vi "Test Process Error on Request Propagated to Caller.vi"(8 "error in (no error)":errorcluster, 11 "Process Test In":refnum<class "Process Dev Test.lvclass">) -> (0 "error out":errorcluster, 3 "Process Test Out":refnum<class "Process Dev Test.lvclass">)   [LabVIEW 2020, in "Process Dev Test.lvclass"]
uses:
  Process Dev Test.lvclass
  Process Dev Test.lvclass/Process Dev Test.ctl
  source/Framework Test Suite/Mock Process/Mock Process.lvclass
  source/Framework/Process/Process.lvclass
  <vilib>/ErrorRing/Error Ring.xnode
  <vilib>/Utility/error.llb/Error Cluster From Error Code.vi
  C:/Git/triarc-framework/source/Framework/Process/Process.lvclass
  C:/Git/triarc-framework/source/Framework/Base/Base.lvclass
  C:/Git/triarc-framework/source/Framework/Configuration File/Configuration File.lvclass
  C:/Git/triarc-framework/source/Framework/Configuration/Configuration.lvclass
  C:/Git/triarc-framework/source/Framework/Error Handler Interface/Error Handler Interface.lvclass
  C:/Git/triarc-framework/source/Framework/Logging/Logging.lvclass
  C:/Git/triarc-framework/source/Framework Test Suite/Mock Process/Mock Process.lvclass
  C:/Git/triarc-framework/source/Framework/Async Handler/Async Handler.lvclass
  C:/Git/triarc-framework/source/Framework/Helper Loop/Helper Loop.lvclass
  <vilib>/Astemes/LUnit/Test Case.lvclass
  C:/Git/triarc-framework/source/Framework Test Suite/Base Class Test/Base Test.lvclass
  C:/Program Files (x86)/National Instruments/LabVIEW 2020/vi.lib/Astemes/LUnit/Test Case.lvclass
  C:/Git/triarc-framework/tests/Process Development Test/Process Test/Process Dev Test.lvclass
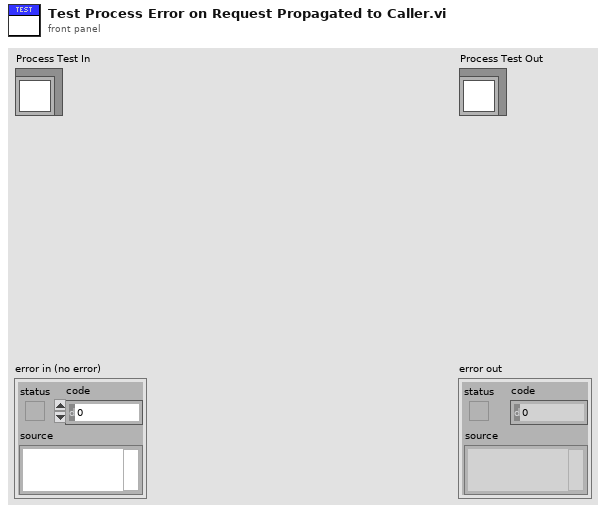
[diagram p1: front panel]
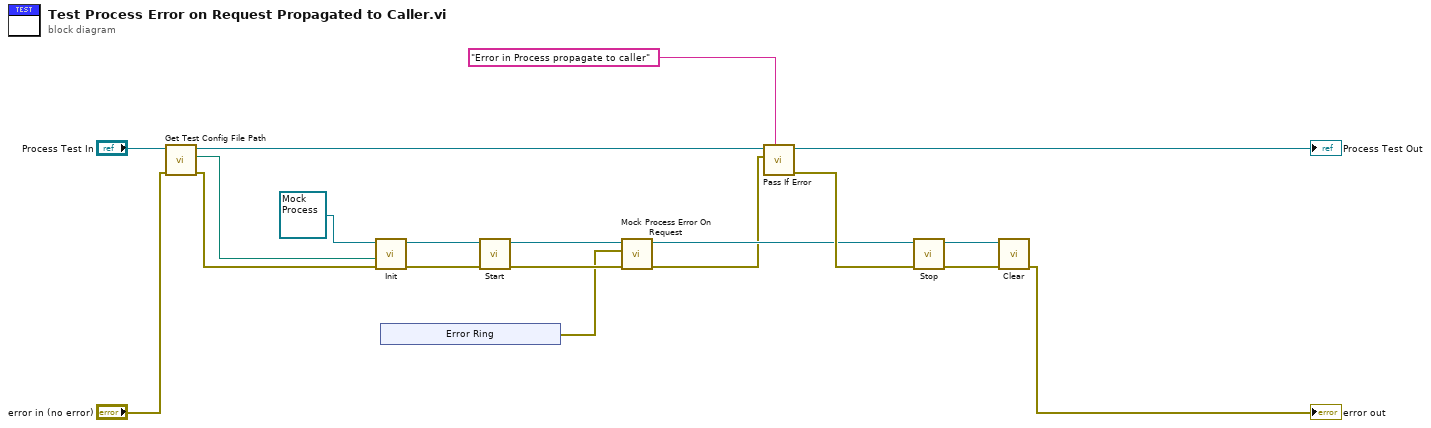
[diagram p0: block diagram]
diagram:
  n1 = call "Get Test Config File Path.vi"("error in (no error)"="error in (no error)", "Process Test In"="Process Test In") -> ("error out"=w13:errorcluster, "Test config path"=w14:path, "Process Test Out"=w2:refnum<class "Process Dev Test.lvclass">)  [unwired: 7 in]
  n2 = call-dynamic "Init.vi"("error in (no error)"=w13, "Config File Path"=w14, "Mock Process In"=refnum<class "Mock Process.lvclass"> refnum ("Mock Process.lvclass")) -> ("error out"=w16:errorcluster, "Mock Process Out"=w17:refnum<class "Mock Process.lvclass">)  [unwired: 7 in]
  n3 = xnode "Error Ring"() -> ("error out"=w6:errorcluster)
  n4 = call "Start.vi"("error in (no error)"=w16, "Process In"=w17) -> ("error out"=w10:errorcluster, "Process Out"=w4:refnum<class "Mock Process.lvclass">)  [unwired: 7 in, 1 out]
  n5 = call "Mock Process Error On Request.vi"("error in (no error)"=w10, "Mock Error"=w6, "Mock Process in"=w4) -> ("error out"=w1:errorcluster, "Mock Process out"=w3:refnum<class "Mock Process.lvclass">)  [unwired: 6 in, 1 out]
  n6 = call <vilib>:"Pass If Error.vi"("Description"="Error in Process propagate to caller", "Assert error"=w1, "LUnit Test Case In"=w2) -> ("error out"=w7:errorcluster, "LUnit Test Case Out"=→"Process Test Out":refnum<class "Process Dev Test.lvclass">)  [unwired: 7 in]
  n7 = call "Stop.vi"("error in (no error)"=w7, "Process In"=w3) -> ("error out"=w5:errorcluster, "Process Out"=w19:refnum<class "Mock Process.lvclass">)  [unwired: 7 in, 1 out]
  n8 = call-dynamic "Clear.vi"("error in (no error)"=w5, "Mock Process In"=w19) -> ("error out"=→"error out":errorcluster)  [unwired: 9 in]
